vi "Default.File.ploy.Add Line to Text Log File.Filepath.vi"(8 "error in (no error)":errorcluster, 10 "Line to Add":string, 11 "Log FilePath":path) -> (0 "error out":errorcluster, 3 "Log FilePath (dup)":path)   [LabVIEW 2010]
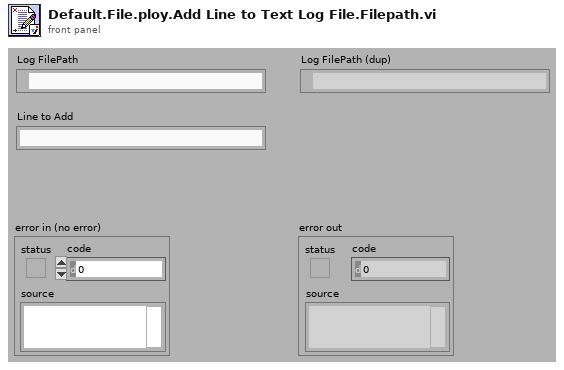
[diagram p1: front panel]
types:
  T1 = enum16{"open", "replace", "create", "open or create", "replace or create", "replace or create with confirmation"}
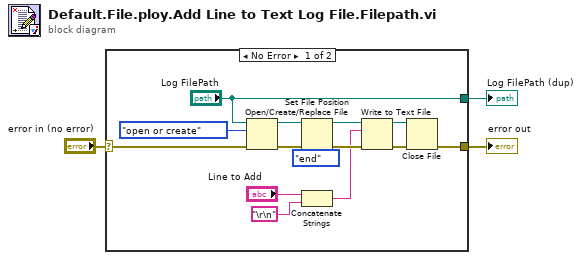
[diagram p0: block diagram]
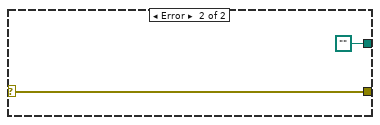
[diagram p2: hidden frame]
diagram:
  n1 = case shown="No Error" "error in (no error)" {
    selector: "error in (no error)" -> [w15 w19]
    tunnel: [w7 w19] -> w3
    tunnel: ["Log FilePath" path ""] -> w1
    frame No Error {
      n2 = Open/Create/Replace File(file path (use dialog)="Log FilePath", error in=w15, operation (0:open)=T1."open or create") -> (refnum out=w13:refnum<file>, error out=w14:errorcluster)  [unwired: 3 in, 1 out]
      n3 = Set File Position(refnum=w13, from (0:start)=enum16{"start", "end", "current"}."end", error in=w14) -> (refnum out=w11:refnum<file>, error out=w12:errorcluster)  [unwired: 1 in]
      n4 = Concatenate Strings("Line to Add", "\r\n") -> (w10:string)
      n5 = Write to Text File(file (use dialog)=w11, text=w10, error in=w12) -> (refnum out=w9:refnum<file>, error out=w8:errorcluster)  [unwired: 1 in, 1 out]
      n6 = Close File(refnum=w9, error in=w8) -> (error out=w7:errorcluster)  [unwired: 1 out]
    }
    frame Error {
    }
  }
  "error out" <- w3
  "Log FilePath (dup)" <- w1
